vi "is color.vi"(10 "Color":T1, 11 "Piece in":refnum<class "Piece.lvclass">) -> (2 "is color?":bool)   [LabVIEW 2015, in "Chesslib.lvlib" / "Piece.lvclass"]
uses:
  Piece.lvclass
  typedef/Color.ctl
  Piece.lvclass/Piece.ctl
  Chesslib.lvlib
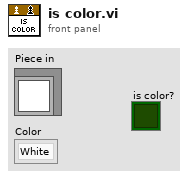
[diagram p1: front panel]
types:
  T1 = typedef "Chesslib.lvlib/Color.ctl" = enum16{"White", "Black"}
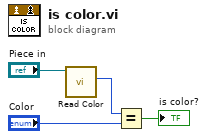
[diagram p0: block diagram]
diagram:
  n1 = call "Read Color.vi"("Piece in"="Piece in") -> ("Color"=w3:T1)  [unwired: 10 in]
  n2 = Equal?(x=w3, y="Color") -> (x = y?=→"is color?":bool)
